vi "1C SmallRCSensorConsole.vi"() -> ()   [LabVIEW 2011]
uses:
  2-RIO/2 Typedefs/Boat Orientation.ctl
  2-RIO/2 Typedefs/Boat Position.ctl
  2-RIO/2 Typedefs/Velocity.ctl
  2-RIO/2 Typedefs/Velocity as Direction and Speed.ctl
panel:
  in  "Add Randomness\nTo Wind Measurement":bool
  out "Simulated\nApparent Wind":T1
  in  "Wind Manual\nInput":T2 {"Direction" scale=0.0..6.283}
  out "Wind Velocity":T1
  out "Boat Velocity":T1
  out "Boat Position":T3
  out "Boat Orientation":T4 scale=0.0..6.283
  out "Overhead Image":T5(plugin-control)
  # "UNFINISHED\nTODO: finish camera interpreter and test!"
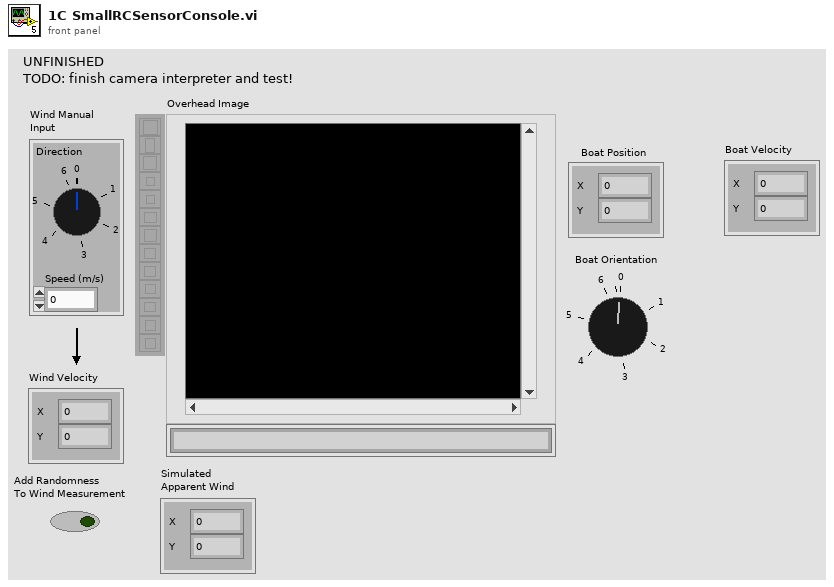
[diagram p1: front panel]
types:
  T1 = typedef "Velocity.ctl" = cluster{"X":dbl, "Y":dbl}
  T2 = typedef "Velocity as Direction and Speed.ctl" = cluster{"Speed (m/s)":dbl, "Direction":dbl}
  T3 = typedef "Boat Position.ctl" = cluster{"X":dbl, "Y":dbl}
  T4 = typedef "Boat Orientation.ctl" = dbl
  T5 = typedef "IMAQ Image.ctl" = refnum<image>
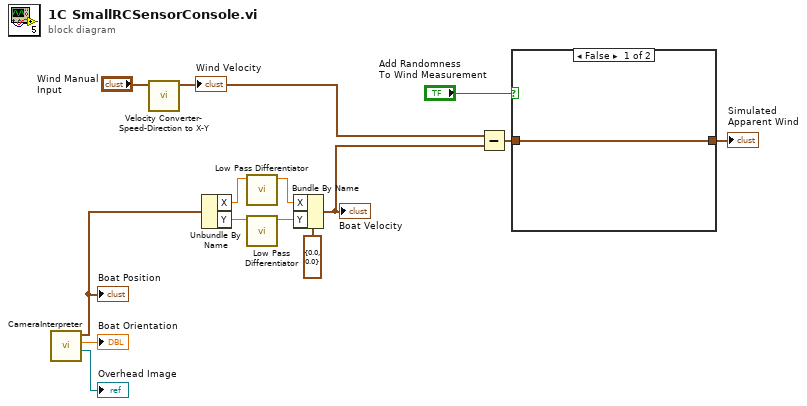
[diagram p0: block diagram]
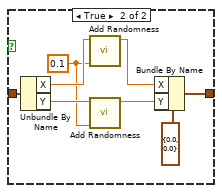
[diagram p2: hidden frame]
diagram:
  n1 = call "CameraInterpreter.vi"() -> ("Overhead Image"=→"Overhead Image":T5, "Boat Orientation"=→"Boat Orientation":T4, "Boat Position"=w12:T3)  [unwired: 9 in]
  "Boat Position" <- w12
  n2 = call "Velocity Converter- Speed-Direction to X-Y.vi"("Velocity as\nDirection/Speed"="Wind Manual\nInput") -> ("Velocity as X/Y"=w4:T1)  [unwired: 10 in]
  "Wind Velocity" <- w4
  n3 = Unbundle By Name(w12) -> ("X"=w11:dbl, "Y"=w10:dbl)
  n4 = call "Low Pass Differentiator.vi"("X"=w11) -> ("dX, smoothed"=w7:dbl)  [unwired: 10 in]
  n5 = call "Low Pass Differentiator.vi"("X"=w10) -> ("dX, smoothed"=w8:dbl)  [unwired: 10 in]
  n6 = Bundle By Name(cluster=T1 {"X"=0.0, "Y"=0.0} ("Boat Velocity 2"), "X"=w7, "Y"=w8) -> (w5:T1)
  "Boat Velocity" <- w5
  n7 = Subtract(x=w4, y=w5) -> (x-y=w2:T1)
  n8 = case shown="False" "Add Randomness\nTo Wind Measurement" {
    tunnel: [w15 w23] -> w3
    tunnel: w2 -> [w15 w21]
    frame False {
    }
    frame True {
      w16 = 0.1 ("Amplitude\n(default 1)")
      n9 = Unbundle By Name(w21) -> ("X"=w20:dbl, "Y"=w19:dbl)
      n10 = call "Add Randomness.vi"("Amplitude\n(default 1)"=w16, "Numeric in"=w20) -> ("Numeric out"=w17:dbl)  [unwired: 9 in]
      n11 = call "Add Randomness.vi"("Amplitude\n(default 1)"=w16, "Numeric in"=w19) -> ("Numeric out"=w18:dbl)  [unwired: 9 in]
      n12 = Bundle By Name(cluster=T1 {"X"=0.0, "Y"=0.0} ("Boat Velocity 2"), "X"=w17, "Y"=w18) -> (w23:T1)
    }
  }
  "Simulated\nApparent Wind" <- w3
